vi "Initialize_Characterization_Tests.vi"(8 "Evnts_per_step":u16, 10 "Free_run_en":bool) -> (0 "Group_Name":string, 2 "error out":errorcluster, 3 "Refnum out":refnum<k34>)   [LabVIEW 2019]
uses:
  SiPM_Tests_Global_Var.vi
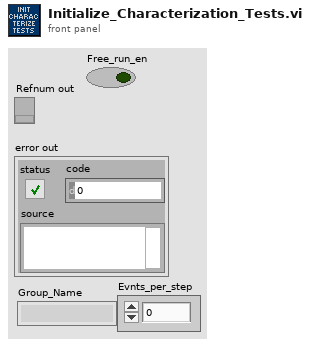
[diagram p1: front panel]
types:
  T1 = enum16{"big-endian, network order", "native, host order", "little-endian"}
  T2 = enum16{"open", "open or create", "create or replace", "create", "open (read-only)"}
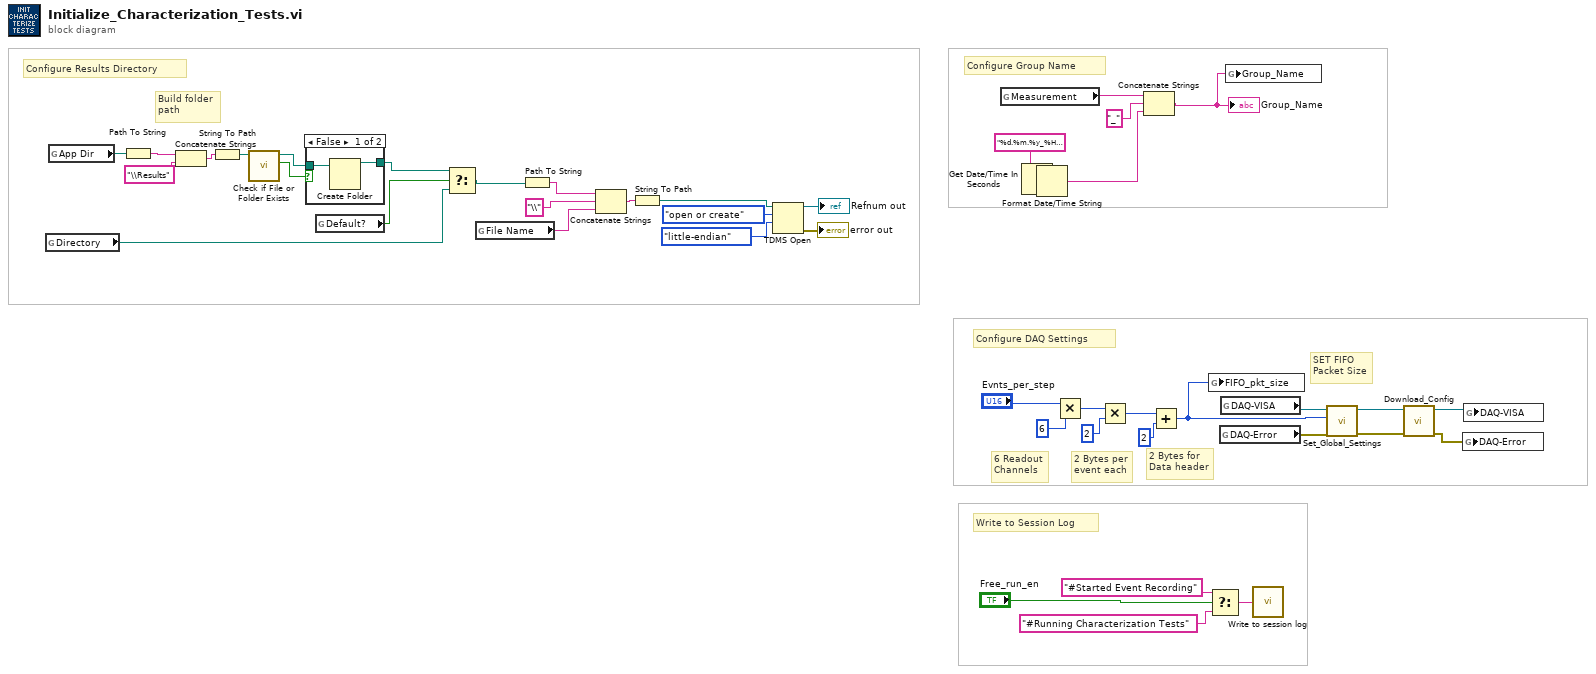
[diagram p0: block diagram]
diagram:
  # "2 Bytes for \nData header"
  # "Configure DAQ Settings"
  # "Write to Session Log"
  # "SET FIFO \nPacket Size"
  # "2 Bytes per\nevent each"
  # "6 Readout\nChannels"
  # "Configure Group Name"
  # "Configure Results Directory"
  # "Build folder\npath"
  n1 = global read "SiPM_Tests_Global_Var.vi" "Directory"() -> (w37:path)
  n2 = global read "SiPM_Tests_Global_Var.vi" "App Dir"() -> (w35:path)
  n3 = Path To String(path=w35) -> (string=w36:string)
  n4 = Concatenate Strings(w36, "\\Results" ("string")) -> (w34:string)
  n5 = String To Path(string=w34) -> (path=w33:path)
  n6 = call <vilib>:"Check if File or Folder Exists.vi"("path"=w33) -> ("file or folder exists?"=w32:bool, "dup path"=w31:path)  [unwired: 8 in, 1 out]
  n7 = case shown="False" w32 {
    tunnel: [w45 w46] -> w38
    tunnel: w31 -> [w44 w46]
    frame False {
      n8 = Create Folder(path (use dialog)=w44) -> (created path=w45:path)  [unwired: 2 in, 2 out]
    }
    frame True {
    }
  }
  n9 = global read "SiPM_Tests_Global_Var.vi" "Default?"() -> (w39:bool)
  n10 = Select(t=w38, s=w39, f=w37) -> (s? t:f=w24:path)
  n11 = global read "SiPM_Tests_Global_Var.vi" "File Name"() -> (w23:string)
  n12 = Path To String(path=w24) -> (string=w26:string)
  n13 = Concatenate Strings(w26, "\\" ("string"), w23) -> (w25:string)
  n14 = String To Path(string=w25) -> (path=w22:path)
  n15 = TDMS Open(9:T1."little-endian" ("byte order (2:little-endian)"), 10:T2."open or create" ("operation (0:open)"), 11:w22) -> (0:→"error out":errorcluster, 3:→"Refnum out":refnum<k34>)  [unwired: 4 in]
  n16 = global read "SiPM_Tests_Global_Var.vi" "Measurement"() -> (w17:string)
  n17 = Get Date/Time In Seconds() -> (seconds since 1Jan1904=w29:timestamp)
  n18 = Format Date/Time String(time format string (%c)="%d.%m.%y_%H.%M_", seconds (now)=w29) -> (date/time string=w15:string)  [unwired: 1 in]
  n19 = Multiply(x="Evnts_per_step", y=u16 6) -> (x*y=w10:u16)
  n20 = Multiply(x=w10, y=u16 2) -> (x*y=w2:u16)
  n21 = Concatenate Strings(w17, "_" ("string"), w15) -> (w4:string)
  "Group_Name" <- w4
  n22 = Add(x=w2, y=u16 2) -> (x+y=w3:u16)
  n23 = global write "SiPM_Tests_Global_Var.vi" "FIFO_pkt_size"(w3) -> ()
  n24 = Select(t="#Started Event Recording" ("Session string"), s="Free_run_en", f="#Running Characterization Tests" ("Session string")) -> (s? t:f=w19:string)
  n25 = global read "SiPM_Tests_Global_Var.vi" "DAQ-Error"() -> (w13:errorcluster)
  n26 = global read "SiPM_Tests_Global_Var.vi" "DAQ-VISA"() -> (w14:refnum<visa-resource-name>)
  n27 = global write "SiPM_Tests_Global_Var.vi" "Group_Name"(w4) -> ()
  n28 = call "Write to session log.vi"("Session string"=w19) -> ()  [unwired: 1 in]
  n29 = call "Set_Global_Settings.vi"("error in (no error)"=w13, "FIFO_PKT_SIZE"=w3, "VISA Refnum in"=w14) -> ("error out"=w7:errorcluster, "VISA Refnum out"=w8:refnum<visa-resource-name>)  [unwired: 7 in]
  n30 = call "Download_Config.vi"("error in"=w7, "VISA in"=w8) -> ("error out"=w5:errorcluster, "VISA Refnum out"=w6:refnum<visa-resource-name>)  [unwired: 8 in]
  n31 = global write "SiPM_Tests_Global_Var.vi" "DAQ-Error"(w5) -> ()
  n32 = global write "SiPM_Tests_Global_Var.vi" "DAQ-VISA"(w6) -> ()
